vi "Actor Core.vi"(8 "error in":errorcluster, 11 "Nested in":refnum<class "DisplayerUI.lvclass">) -> (0 "error out":errorcluster, 3 "Actor out":refnum<class "Actor.lvclass">)   [LabVIEW 2020, in "Displayer.lvlib" / "DisplayerUI.lvlib" / "DisplayerUI.lvclass"]
doc: "(<B>Filename</B>: Actor Framework.lvlib:Actor.lvclass:Actor Core.vi)\n\nReceives messages to the actor, reacts to them, and initiates any error handling that may shut the actor down.\n\nDescendant classes may override this VI to append parallel tasks for the actor to complete while it handles messages. Overrides use the Call Parent Method node."
uses:
  DisplayerUI.lvclass
  C:/Program Files/National Instruments/LabVIEW 2020/vi.lib/ActorFramework/Actor/Actor.lvclass
  <vilib>/ActorFramework/Actor/Actor.lvclass
  DisplayerUI.lvclass/DisplayerUI.ctl
  <vilib>/ActorFramework/Actor/Actor.lvclass/Actor.ctl
  <vilib>/ActorFramework/Message Enqueuer/Message Enqueuer.lvclass/Message Enqueuer.ctl
  Displayer/Displayer Messages/ImageMouseWheel Msg/ImageMouseWheel Msg.lvclass/ImageMouseWheel Msg.ctl
  DisplayerUI Messages/PrepareAndSendSetROI Msg/PrepareAndSendSetROI Msg.lvclass/PrepareAndSendSetROI Msg.ctl
  <vilib>/Utility/miscctls.llb/LVRangeTypeDef.ctl
  <vilib>/ActorFramework/Message Enqueuer/Init from Existing Queue.vi
  <vilib>/ActorFramework/Message Enqueuer/Enqueue.vi
  Displayer/Displayer Messages/ImageMouseWheel Msg/ImageMouseWheel Msg.lvclass
  C:/Program Files/National Instruments/LabVIEW 2020/vi.lib/ActorFramework/Message/Message.lvclass
  DisplayerUI Messages/PrepareAndSendSetROI Msg/PrepareAndSendSetROI Msg.lvclass
  <vilib>/ActorFramework/Stop Msg/Stop Msg.lvclass
  <vilib>/ActorFramework/Message Priority Queue/Priority Enqueue.vi
  <vilib>/ActorFramework/Message Enqueuer/Message Enqueuer.lvclass
panel:
  out "Max":dbl
  out "Min":dbl
  in  "Display Max":dbl
  in  "Display Min":dbl
  out "ImgIndex":dbl
  out "FPS":dbl
  in  "Threshold":cluster{i16, i16}(slide)={500, 0} scale=0.0..4096.0
  in  "Autostretch":bool
  in  "ZoomToFit":bool
  in  "Full":bool
  in  "Crop":bool
  in  "Scale Bar":bool
  in  "ScaleBarSize":dbl caption="um" min=0.0 max=50.0
  out "RawImage":T1(plugin-control)
  # "-"
  # "-"
  # "Display Range"
  # "TH"
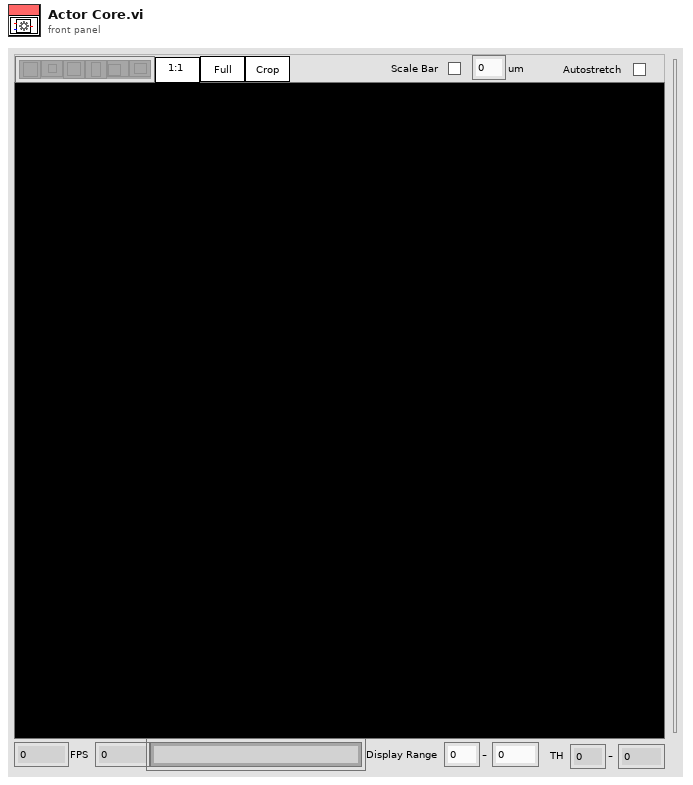
[diagram p1: front panel]
types:
  T1 = typedef "IMAQ Image.ctl" = refnum<image>
  T2 = cluster{"Stop":refnum<user-event>, "DisplayImage":refnum<user-event>}
  T3 = cluster{"Global Rectangle":i32[], "Contours":cluster{"Contour Type":u32, "ROI Type":u32, "Points":i32[]}[]}
  T4 = typedef "LVRangeTypeDef.ctl" = cluster{"Minimum":dbl, "Maximum":dbl, "Increment":dbl, "Minor Increment":dbl, "Start":dbl}
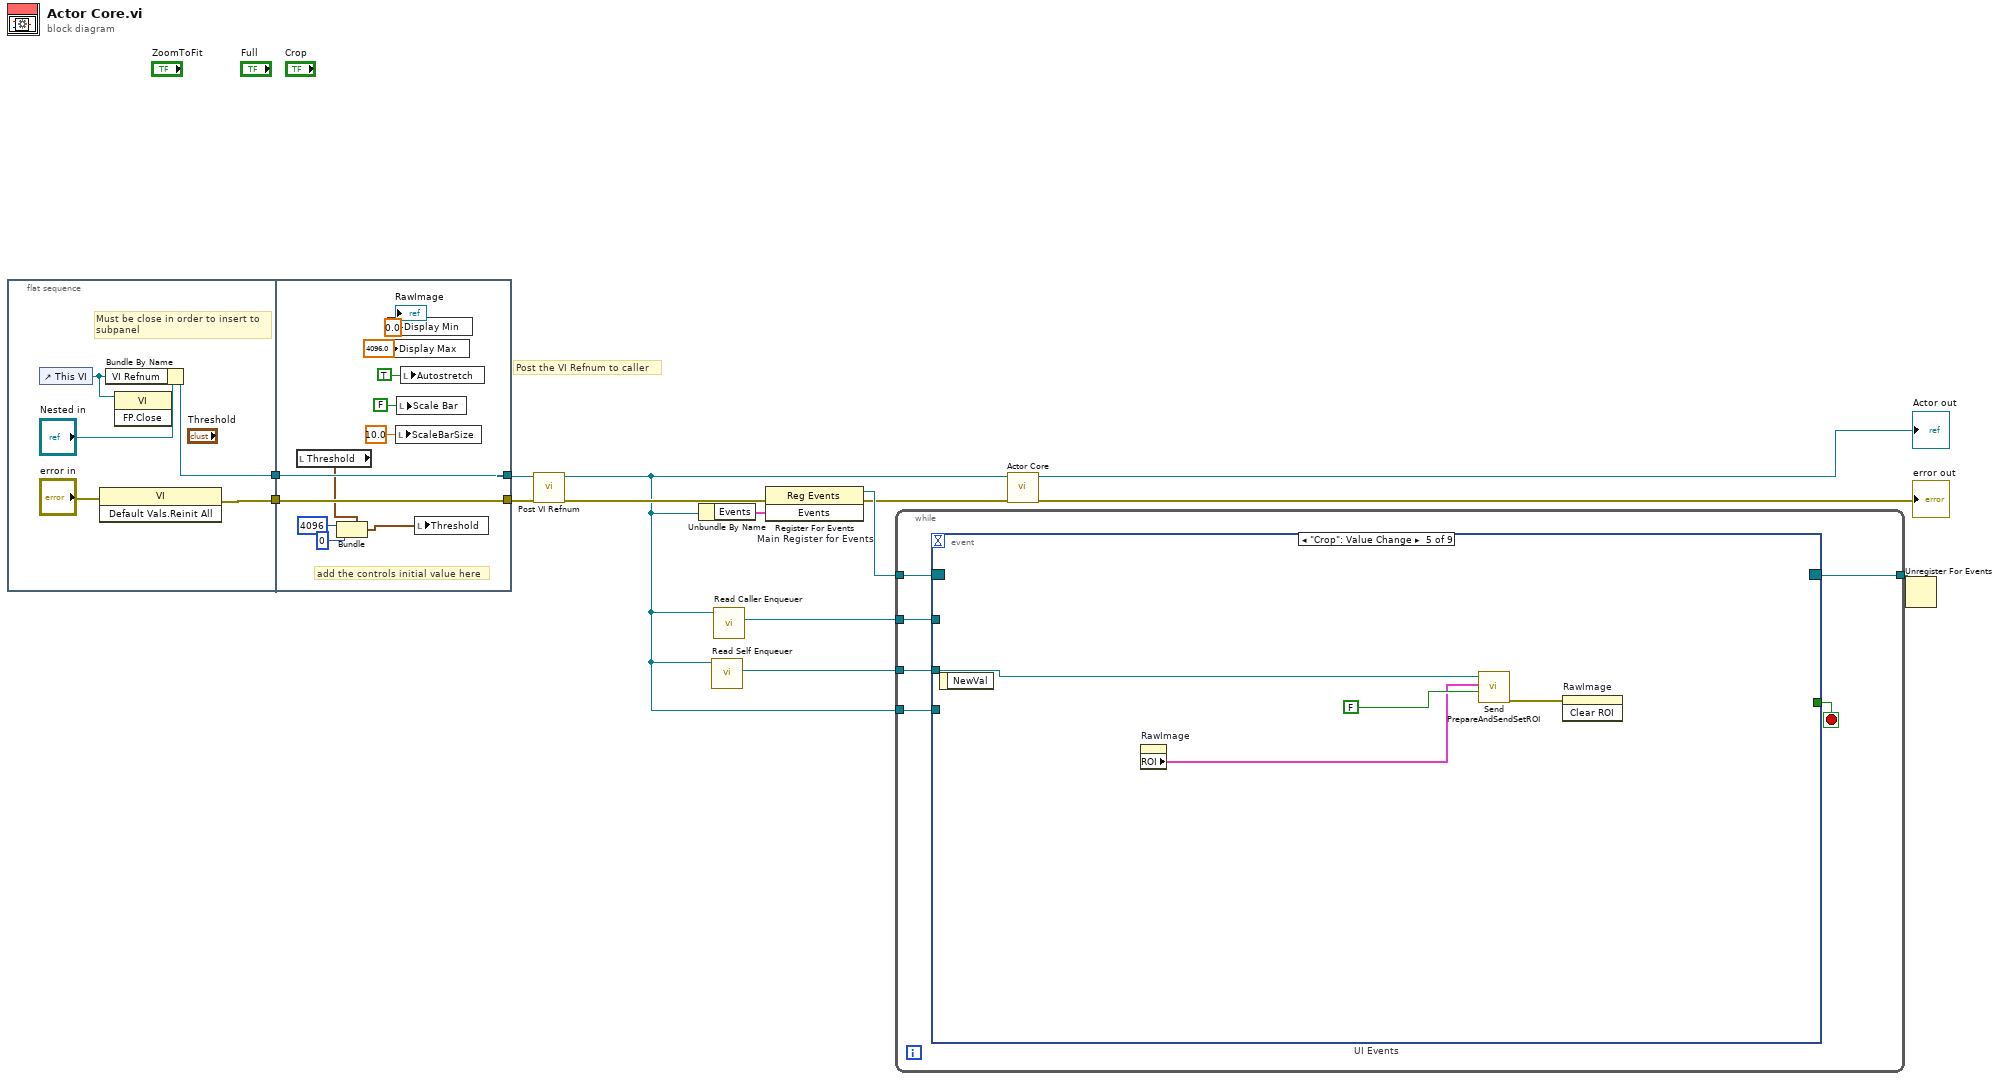
[diagram p0: block diagram]
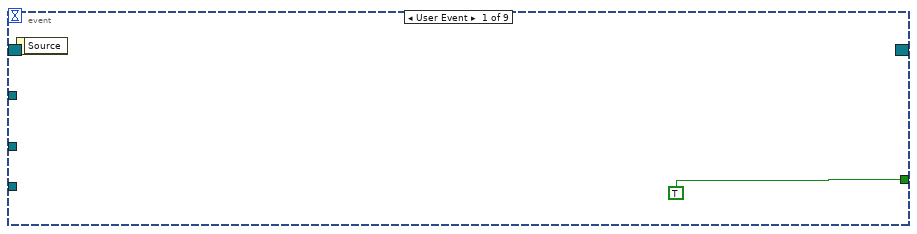
[diagram p2: hidden frame]
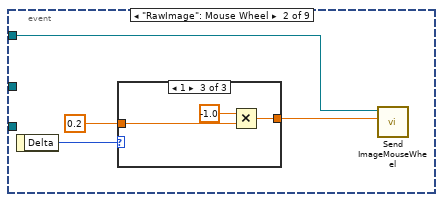
[diagram p3: hidden frame]
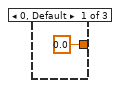
[diagram p4: hidden frame]
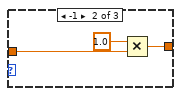
[diagram p5: hidden frame]
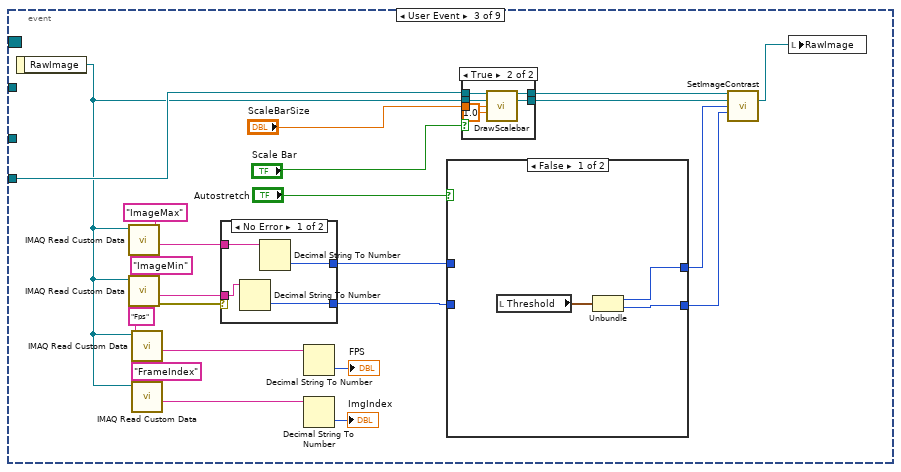
[diagram p6: hidden frame]
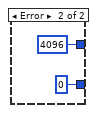
[diagram p7: hidden frame]
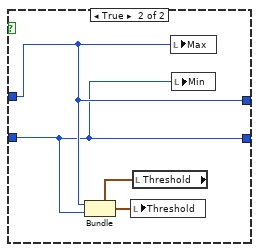
[diagram p8: hidden frame]
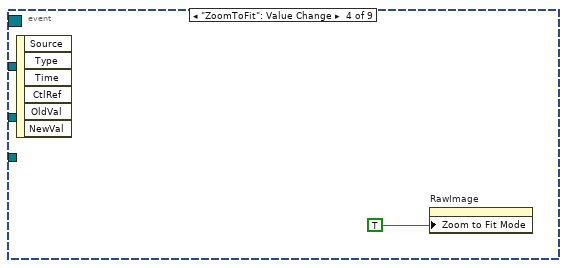
[diagram p10: hidden frame]
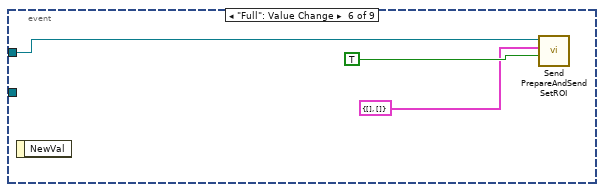
[diagram p11: hidden frame]
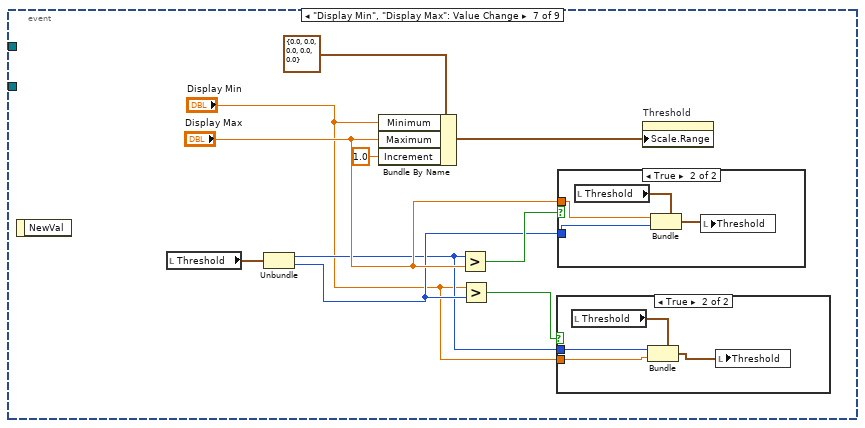
[diagram p12: hidden frame]
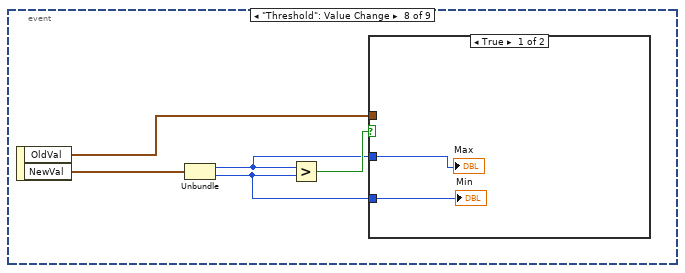
[diagram p15: hidden frame]
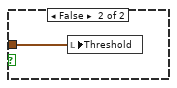
[diagram p16: hidden frame]
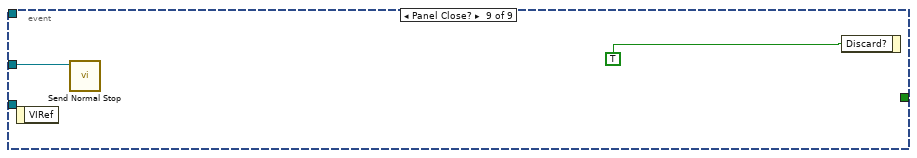
[diagram p17: hidden frame]
diagram:
  # "Post the VI Refnum to caller"
  n1 = flat-sequence {
    tunnel: [w17] -> w6
    tunnel: [w16] -> w5
    tunnel: [w29] -> w3
    tunnel: [w30] -> w7
    tunnel: w6 -> [w30]
    tunnel: w5 -> [w29]
    frame #0 {
      # "Must be close in order to insert to\nsubpanel"
      n2 = control-ref of="This VI"() -> (w15:refnum<vi>)
      n3 = invoke class="VI" method="Default Vals.Reinit All"(error in="error in") -> (error out=w17:errorcluster)  [unwired: 2 in, 2 out]
      n4 = Bundle By Name(cluster="Nested in", "VI Refnum"=w15) -> (w16:refnum<class "DisplayerUI.lvclass">)
      n5 = invoke class="VI" method="FP.Close"(reference=w15) -> ()  [unwired: 2 in, 3 out]
    }
    frame #1 {
      # "add the controls initial value here"
      n6 = local read "Threshold"() -> (w24:cluster{i16, i16})
      n7 = Bundle(cluster=w24, i16 4096, i16 0) -> (w25:cluster{i16, i16})
      n8 = local write "Display Max"(4096.0 ("Max")) -> ()
      n9 = local write "Display Min"(0.0 ("Min")) -> ()
      n10 = local write "ScaleBarSize"(10.0 ("ScaleBarSize")) -> ()
      n11 = local write "Scale Bar"(FALSE ("Scale Bar")) -> ()
      n12 = local write "Autostretch"(TRUE ("Autostretch")) -> ()
      n13 = local write "Threshold"(w25) -> ()
    }
  }
  n14 = call-dynamic "Post VI Refnum.vi"("error in (no error)"=w7, "Controller Template in"=w3) -> ("error out"=w4:errorcluster, "Controller Template out"=w1:refnum<class "DisplayerUI.lvclass">)  [unwired: 8 in]
  n15 = Unbundle By Name(w1) -> ("Events"=w11:T2)
  n16 = call <vilib>:"Read Self Enqueuer.vi"("Actor"=w1) -> ("Self Enqueuer"=w9:refnum<class "Message Enqueuer.lvclass">)  [unwired: 10 in]
  n17 = call <vilib>:"Read Caller Enqueuer.vi"("Actor"=w1) -> ("Caller Enqueuer"=w2:refnum<class "Message Enqueuer.lvclass">)  [unwired: 10 in]
  n18 = register-events "Main Register for Events"(error in=w4, w11) -> (reference out=w12:refnum<event-registration>, error out=w8:errorcluster)  [unwired: 1 in]
  n19 = while {
    tunnel: w12 -> [w36]
    tunnel: [w34] -> w10
    tunnel: w9 -> [w33]
    tunnel: w2 -> [w32]
    tunnel: w1 -> [w31]
    stop <- w35 stop-if-true
    n20 = event "UI Events" shown="[4] \"Crop\": Value Change" {
      selector: w36 -> [_ _ _ _ _ _ _ _ _]
      dyn-events: [_ _ _ _ _ _ _ _ _] -> w34
      timeout: _ -> [_ _ _ _ _ _ _ _ _]
      tunnel: [TRUE _ _ _ _ _ _ _ _] -> w35
      tunnel: w33 -> [_ _ _ _ w94 w98 _ _ w127]
      tunnel: w32 -> [_ w38 _ _ _ _ _ _ _]
      tunnel: w31 -> [_ _ w52 _ _ _ _ _ _]
      event User Event {
        n21 = event-data() -> ()  [unwired: 1 in, 1 out]
      }
      event "RawImage": Mouse Wheel {
        n22 = event-data() -> ("Delta"=w40:i32)  [unwired: 1 in]
        n23 = case shown="1" w40 {
          tunnel: 0.2 ("Value") -> [_ w45 w48]
          tunnel: [0.0 w43 w46] -> w39
          frame 0, Default {
          }
          frame -1 {
            n24 = Multiply(x=1.0, y=w45) -> (x*y=w43:dbl)
          }
          frame 1 {
            n25 = Multiply(x=-1.0, y=w48) -> (x*y=w46:dbl)
          }
        }
        n26 = call "Send ImageMouseWheel.vi"("Value"=w39, "Message Enqueuer"=w38) -> ()  [unwired: 8 in, 2 out]
      }
      event User Event {
        n27 = event-data() -> ("RawImage"=w51:T1)  [unwired: 1 in]
        n28 = call "IMAQ Read Custom Data"("Key"="ImageMax", "Image"=w51) -> ("Custom Data Out"=w56:string)  [unwired: 7 in, 2 out]
        n29 = call "IMAQ Read Custom Data"("Key"="ImageMin", "Image"=w51) -> ("error out"=w55:errorcluster, "Custom Data Out"=w57:string)  [unwired: 7 in, 1 out]
        n30 = call "IMAQ Read Custom Data"("Key"="Fps", "Image"=w51) -> ("Custom Data Out"=w70:string)  [unwired: 7 in, 2 out]
        n31 = call "IMAQ Read Custom Data"("Key"="FrameIndex", "Image"=w51) -> ("Custom Data Out"=w67:string)  [unwired: 7 in, 2 out]
        n32 = case shown="No Error" w55 {
          tunnel: w57 -> [w75 _]
          tunnel: w56 -> [w74 _]
          tunnel: [w72 0] -> w49
          tunnel: [w73 4096] -> w50
          frame No Error {
            n33 = Decimal String To Number(string=w75) -> (number=w72:i32)  [unwired: 2 in, 1 out]
            n34 = Decimal String To Number(string=w74) -> (number=w73:i32)  [unwired: 2 in, 1 out]
          }
          frame Error {
          }
        }
        n35 = Decimal String To Number(string=w70) -> (number=→"FPS":i32)  [unwired: 2 in, 1 out]
        n36 = Decimal String To Number(string=w67) -> (number=→"ImgIndex":i32)  [unwired: 2 in, 1 out]
        n37 = case shown="False" "Autostretch" {
          tunnel: [w79 w82] -> w61
          tunnel: [w78 w81] -> w60
          tunnel: w50 -> [_ w82]
          tunnel: w49 -> [_ w81]
          frame False {
            n38 = local read "Threshold"() -> (w80:cluster{i16, i16})
            n39 = Unbundle(w80) -> (w79:i16, w78:i16)
          }
          frame True {
            n40 = local read "Threshold"() -> (w84:cluster{i16, i16})
            n41 = Bundle(cluster=w84, w82, w81) -> (w83:cluster{i16, i16})
            n42 = local write "Threshold"(w83) -> ()
            n43 = local write "Max"(w82) -> ()
            n44 = local write "Min"(w81) -> ()
          }
        }
        n45 = case shown="True" "Scale Bar" {
          tunnel: w52 -> [w86 w92]
          tunnel: [w86 w91] -> w63
          tunnel: w51 -> [w85 w90]
          tunnel: [w85 w89] -> w62
          tunnel: "ScaleBarSize" -> [_ w88]
          frame False {
          }
          frame True {
            n46 = call-dynamic "DrawScalebar.vi"("DisplayerUI in"=w92, "Image In"=w90, "ScaleBarSize"=w88, "Binning"=1.0) -> ("DisplayerUI out"=w91:refnum<class "DisplayerUI.lvclass">, "Image Out"=w89:T1)  [unwired: 9 in, 1 out]
          }
        }
        n47 = call-dynamic "SetImageContrast.vi"("DisplayerUI in"=w63, "Image In"=w62, "Max"=w61, "Min"=w60) -> ("Image Dst Out"=w59:T1)  [unwired: 9 in, 2 out]
        n48 = local write "RawImage"(w59) -> ()
      }
      event "ZoomToFit": Value Change {
        n49 = event-data() -> ()  [unwired: 1 in, 6 out]
        n50 = property on="RawImage" class="ImageControl"("Zoom to Fit Mode"=TRUE) -> ()  [unwired: 2 in, 2 out]
      }
      event "Crop": Value Change {
        n51 = event-data() -> ()  [unwired: 1 in, 1 out]
        n52 = property on="RawImage" class="ImageControl"() -> ("ROI"=w96:T3)  [unwired: 2 in, 2 out]
        n53 = call "Send PrepareAndSendSetROI.vi"("Clear ROI?(F)"=FALSE, "ROI"=w96, "Message Enqueuer"=w94) -> ("error out"=w95:errorcluster)  [unwired: 7 in, 1 out]
        n54 = invoke on="RawImage" class="ImageControl" method="Clear ROI"(error in=w95) -> ()  [unwired: 2 in, 3 out]
      }
      event "Full": Value Change {
        n55 = event-data() -> ()  [unwired: 1 in, 1 out]
        n56 = call "Send PrepareAndSendSetROI.vi"("Clear ROI?(F)"=TRUE, "ROI"=T3 {"Global Rectangle"=[], "Contours"=[]}, "Message Enqueuer"=w98) -> ()  [unwired: 7 in, 2 out]
      }
      event "Display Min", "Display Max": Value Change {
        n57 = event-data() -> ()  [unwired: 1 in, 1 out]
        n58 = local read "Threshold"() -> (w107:cluster{i16, i16})
        n59 = Unbundle(w107) -> (w102:i16, w103:i16)
        n60 = Bundle By Name(cluster=T4 {"Minimum"=0.0, "Maximum"=0.0, "Increment"=0.0, "Minor Increment"=0.0, "Start"=0.0} ("Scale.Range"), "Minimum"="Display Min", "Maximum"="Display Max", "Increment"=1.0) -> (w109:T4)
        n61 = Greater?(x=w102, y="Display Max") -> (0:w106:bool)
        n62 = Greater?(x="Display Min", y=w103) -> (0:w105:bool)
        n63 = case shown="True" w105 {
          tunnel: w102 -> [_ w112]
          tunnel: "Display Min" -> [_ w111]
          frame False {
          }
          frame True {
            n64 = local read "Threshold"() -> (w114:cluster{i16, i16})
            n65 = Bundle(cluster=w114, w112, w111) -> (w113:cluster{i16, i16})
            n66 = local write "Threshold"(w113) -> ()
          }
        }
        n67 = case shown="True" w106 {
          tunnel: "Display Max" -> [_ w116]
          tunnel: w103 -> [_ w115]
          frame False {
          }
          frame True {
            n68 = local read "Threshold"() -> (w118:cluster{i16, i16})
            n69 = Bundle(cluster=w118, w116, w115) -> (w117:cluster{i16, i16})
            n70 = local write "Threshold"(w117) -> ()
          }
        }
        n71 = property on="Threshold" class="Slide (strict)"("Scale.Range"=w109) -> ()  [unwired: 2 in, 2 out]
      }
      event "Threshold": Value Change {
        n72 = event-data() -> ("OldVal"=w121:cluster{i16, i16}, "NewVal"=w123:cluster{i16, i16})  [unwired: 1 in]
        n73 = Unbundle(w123) -> (w120:i16, w119:i16)
        n74 = Greater?(x=w120, y=w119) -> (0:w122:bool)
        n75 = case shown="True" w122 {
          tunnel: w121 -> [_ w126]
          tunnel: w120 -> [w125 _]
          tunnel: w119 -> [w124 _]
          frame True {
            "Min" <- w124
            "Max" <- w125
          }
          frame False {
            n76 = local write "Threshold"(w126) -> ()
          }
        }
      }
      event Panel Close? {
        n77 = event-data() -> ()  [unwired: 1 in, 1 out]
        n78 = call <vilib>:"Send Normal Stop.vi"("Message Enqueuer"=w127) -> ()  [unwired: 10 in, 1 out]
        n79 = event-data("Discard?"=TRUE) -> ()  [unwired: 1 in, 1 out]
      }
    }
  }
  n80 = call-parent "Actor Core.vi"("error in"=w8, "Actor in"=w1) -> ("error out"=→"error out":errorcluster, "Actor out"=→"Actor out":refnum<class "Actor.lvclass">)  [unwired: 8 in]
  n81 = Unregister For Events(event registration refnum=w10) -> ()  [unwired: 1 in, 1 out]
